vi "IIR Filter.vi"   [LabVIEW 2024, in "NI_AALBase.lvlib"]
doc: "<p>Filters the input sequence <strong>X</strong> using the direct form IIR filter specified by <strong>Reverse Coefficients</strong> and <strong>Forward Coefficients</strong>. Wire data to the <strong>X</strong> input to determine the polymorphic instance to use or <a href=\"nihelplauncher://docs/csh?context=lvcore_lvhowto_selectingdefaultinstpolyvi\">manually select</a> the instance.\n</p>"
uses:
  NI_AALBase.lvlib
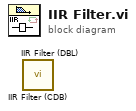
[diagram p0: block diagram]
diagram:
  n1 = call "IIR Filter (CDB).vi"() -> ()  [unwired: 4 in, 2 out]
  n2 = call "IIR Filter (DBL).vi"() -> ()  [unwired: 4 in, 2 out]
